vi "LcWebView_LinePlot_Example.vi"() -> ()   [LabVIEW 2018, in "LcWebView.lvclass"]
doc: "Inject javascript arguments"
uses:
  LcWebView.lvclass
  plots/ctrls/PlotType.ctl
  plots/ctrls/GenericPlotOption.ctl
  plots/ctrls/LegendPosition.ctl
  plots/ctrls/LinePlotOption.ctl
  C:/Projects/LcWebView2/LcWebView/LcWebView_class/data/Microsoft.Web.WebView2.WinForms.dll
  data/Microsoft.Web.WebView2.WinForms.dll
panel:
  out "BrowserProcessId":u32
  out "Status Message":string
  in  "stop":bool
  in  "Web":refnum<k24>(container)
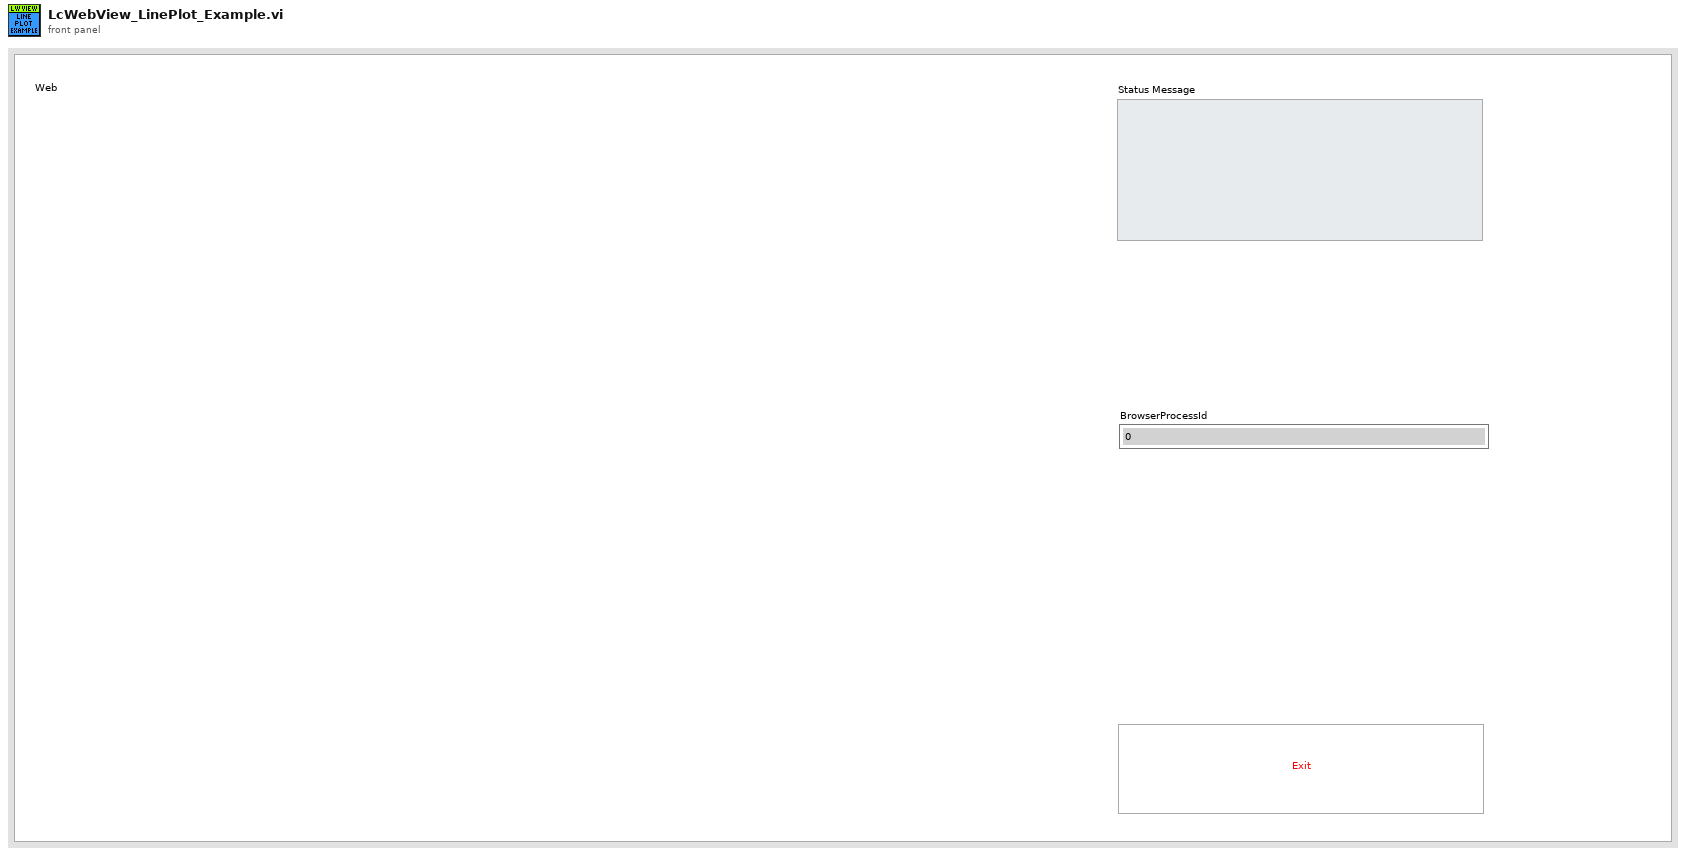
[diagram p1: front panel]
types:
  T1 = typedef "LcWebView.lvclass/GenericPlotOption.ctl" = cluster{"GraphTitle":string, "LegendDisplay":bool, "LegendPosition":T2}
  T2 = typedef "LcWebView.lvclass/LegendPosition.ctl" = enum16{"top", "right", "left", "bottom"}
  T3 = typedef "LcWebView.lvclass/LinePlotOption.ctl" = cluster{"xLabel":string, "yLabel":string, "DisplayXLabel":bool, "DisplayYLabel":bool}
  T4 = typedef "LcWebView.lvclass/PlotType.ctl" = enum16{"bar", "line", "pie", "doughnut", "scatter", "radar", "bubble", "polarArea"}
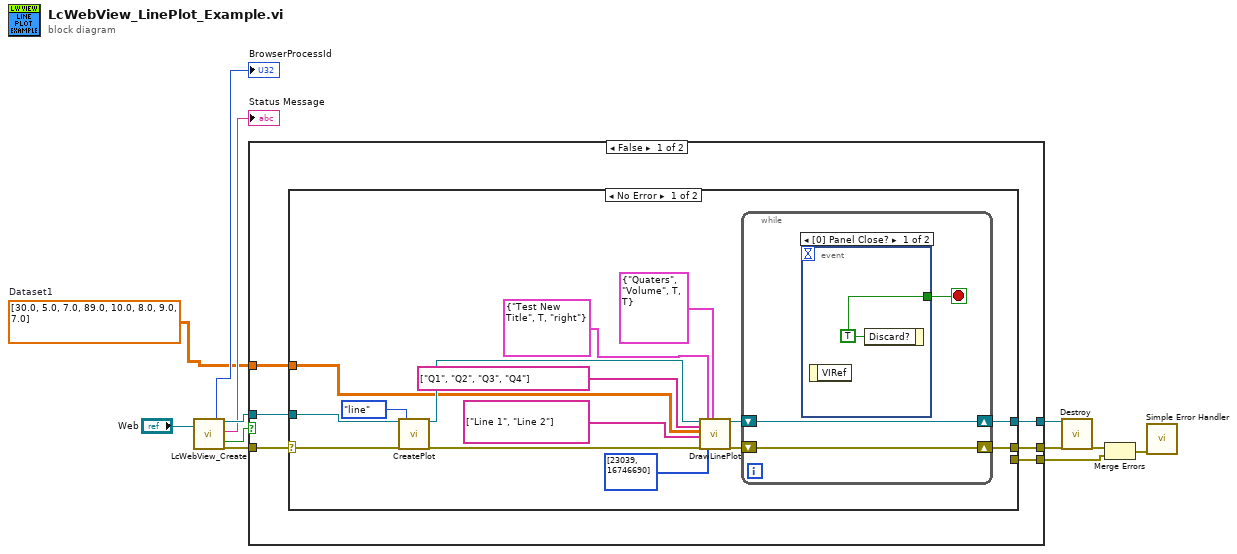
[diagram p0: block diagram]
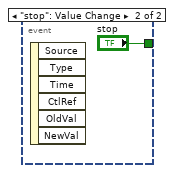
[diagram p2: hidden frame]
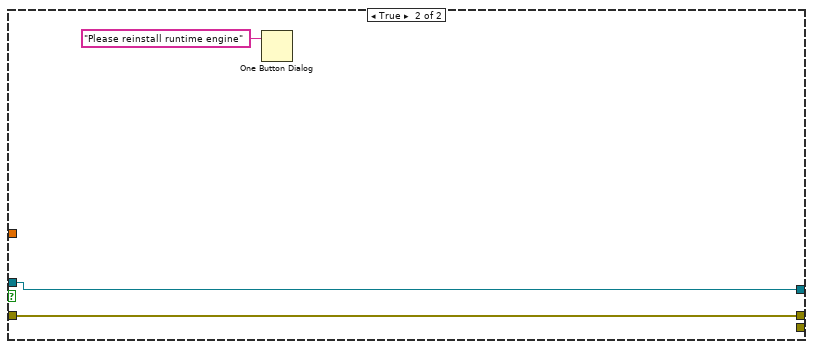
[diagram p4: hidden frame]
diagram:
  w1 = dbl[][] [[30.0, 5.0, 7.0, 89.0], [10.0, 8.0, 9.0, 7.0]]  # Dataset1
  n1 = call "LcWebView_Create.vi"("Webview container"="Web") -> ("BrowserProcessId"=→"BrowserProcessId":u32, "reference out"=w11:refnum<class "LcWebView.lvclass">, "Status Message"=→"Status Message":string, "Reinstall Runtime"=w4:bool, "Error Out"=w10:errorcluster)  [unwired: 11 in, 3 out]
  n2 = case shown="False" w4 {
    tunnel: w11 -> [w18 w43]
    tunnel: w10 -> [w17 w42]
    tunnel: [w16 w43] -> w9
    tunnel: [w14 w42] -> w8
    tunnel: [w15 _] -> w5
    tunnel: w1 -> [w13 _]
    frame False {
      n3 = case shown="No Error" w17 {
        selector: w17 -> [w31 w39]
        tunnel: w18 -> [w32 w40]
        tunnel: [w30 w40] -> w16
        tunnel: [w33 _] -> w14
        tunnel: [_ w39] -> w15
        tunnel: w13 -> [w28 _]
        frame No Error {
          n4 = call-dynamic "CreatePlot.vi"("reference in"=w32, "Error In"=w31, "PlotType"=PlotType."line") -> ("reference out"=w29:refnum<class "LcWebView.lvclass">, "Error Out"=w25:errorcluster)  [unwired: 15 in]
          n5 = call-dynamic "DrawLinePlot.vi"("reference in"=w29, "XLabels"=string[] ["Q1", "Q2", "Q3", "Q4"], "LinePlot.Dataset"=w28, "LinePlot.DatasetLabels"=string[] ["Line 1", "Line 2"] ("DatasetLabels"), "Error In"=w25, "GenericPlotOptions"=T1 {"GraphTitle"="Test New Title", "LegendDisplay"=TRUE, "LegendPosition"=enum."right"}, "BarPlot.PlotColours"=u32[] [23039, 16746690] ("PlotColours"), "BarPlotOptions"=T3 {"xLabel"="Quaters", "yLabel"="Volume", "DisplayXLabel"=TRUE, "DisplayYLabel"=TRUE}) -> ("reference out"=w27:refnum<class "LcWebView.lvclass">, "Error Out"=w26:errorcluster)  [unwired: 10 in]
          n6 = while {
            shift-right: [w36] -> w30
            shift-left: w27 -> [w36]
            shift-right: [w35] -> w33
            shift-left: w26 -> [w35]
            stop <- w34 stop-if-true
            n7 = event shown="[0] Panel Close?" {
              selector: _ -> [_ _]
              dyn-events: _ -> [_ _]
              timeout: _ -> [_ _]
              tunnel: [w37 "stop"] -> w34
              event Panel Close? {
                w37 = TRUE ("Discard?")
                n8 = event-data() -> ()  [unwired: 1 in, 1 out]
                n9 = event-data("Discard?"=w37) -> ()  [unwired: 1 in, 1 out]
              }
              event "stop": Value Change {
                n10 = event-data() -> ()  [unwired: 1 in, 6 out]
              }
            }
          }
        }
        frame Error {
        }
      }
    }
    frame True {
      n11 = One Button Dialog(message="Please reinstall runtime engine") -> ()  [unwired: 1 in, 1 out]
    }
  }
  n12 = call-dynamic "Destroy.vi"("reference in"=w9, "Error In"=w8) -> ("Error Out"=w7:errorcluster)  [unwired: 16 in, 1 out]
  n13 = Merge Errors(w7, w5) -> (w2:errorcluster)
  n14 = call <vilib>:"Simple Error Handler.vi"("error in (no error)"=w2) -> ()  [unwired: 4 in, 5 out]
